vi "U2044XA Measure RF Power.vi"(4 "Route Names":string[](array[string]), 6 "Pwr Mtr Cal":bool=TRUE, 8 "error in":errorcluster, 10 "Input parameters":T1={"Channel (1)"=1, "Avg Count"=4, "Correction Frequency"=50000000.0, "Delay(ms)"=10000, "Reset Device"=FALSE, "ID Query"=FALSE, "Resource Name"="USB0::0x2A8D::0x1E01::MY58390008::INSTR", "Ref Level (dB)"=20.0} {"Ref Level (dB)" format="%^.2e"; "Correction Frequency" format="%.2p"}, 11 "VISA session":refnum<visa-resource-name>="PM2") -> (0 "error out":errorcluster, 2 "dBm":dbl format="%.5f", 3 "dup VISA session":refnum<visa-resource-name>)   [LabVIEW 2015]
doc: "This VI runs one sensor measurement.\n- Open session to sensor specified by Resource Name\n- Sets correct frequency\n- Initialize acqusistion, wait specified time for measurement and reads it."
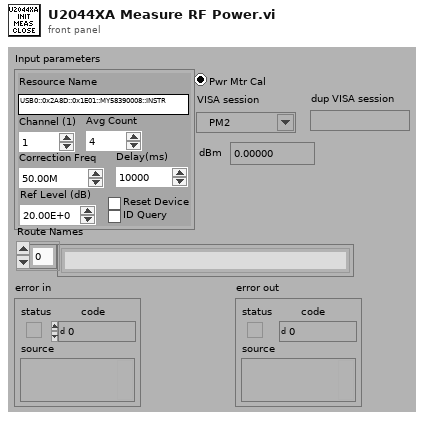
[diagram p1: front panel]
types:
  T1 = cluster{"Channel (1)":i32, "Avg Count":i32, "Correction Frequency":dbl, "Delay(ms)":u32, "Reset Device":bool, "ID Query":bool, "Resource Name":string, "Ref Level (dB)":dbl}
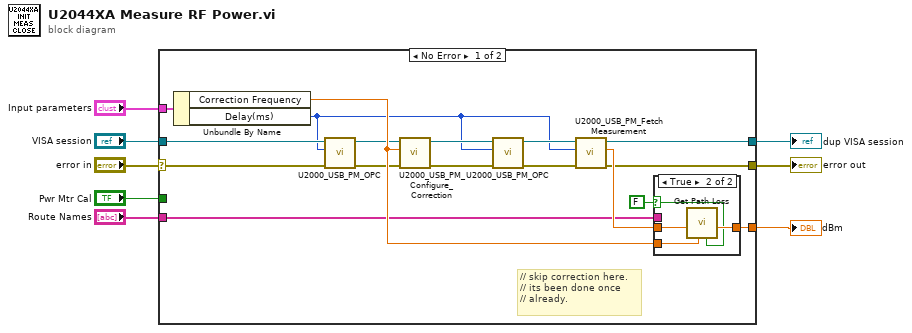
[diagram p0: block diagram]
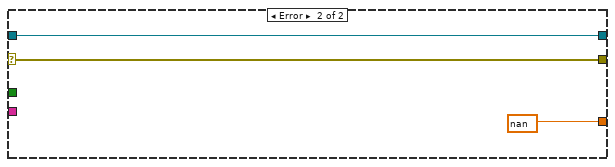
[diagram p3: hidden frame]
diagram:
  n1 = case shown="No Error" "error in" {
    selector: "error in" -> [w16 w33]
    tunnel: [w23 w33] -> w7
    tunnel: "Input parameters" -> [w22 _]
    tunnel: "VISA session" -> [w17 w32]
    tunnel: [w21 w32] -> w4
    tunnel: "Route Names" -> [w20 _]
    tunnel: "Pwr Mtr Cal" -> [_ _]
    tunnel: [w19 nan ("Adjusted Power Level")] -> w1
    frame No Error {
      # "// skip correction here.\n// its been done once\n// already."
      n2 = Unbundle By Name(w22) -> ("Correction Frequency"=w25:dbl, "Delay(ms)"=w9:u32)
      n3 = call "U2000_USB_PM_OPC.vi"("error in (no error)"=w16, "Wait (100ms)"=w9, "VISA resource name"=w17) -> ("error out"=w15:errorcluster, "VISA resource name out"=w14:refnum<visa-resource-name>)  [unwired: 7 in]
      n4 = call "U2000_USB_PM_Configure_Correction.vi"("error in (no error)"=w15, "Frequency (5E+7 Hz)"=w25, "VISA resource name"=w14) -> ("error out"=w13:errorcluster, "VISA resource name out"=w11:refnum<visa-resource-name>)  [unwired: 7 in]
      n5 = call "U2000_USB_PM_OPC.vi"("error in (no error)"=w13, "Wait (100ms)"=w9, "VISA resource name"=w11) -> ("error out"=w12:errorcluster, "VISA resource name out"=w10:refnum<visa-resource-name>)  [unwired: 7 in]
      n6 = call "U2000_USB_PM_Fetch Measurement.vi"("error in (no error)"=w12, "Timeout (10000 ms)"=w9, "VISA resource name"=w10) -> ("error out"=w23:errorcluster, "Measurement"=w24:dbl, "VISA resource name out"=w21:refnum<visa-resource-name>)  [unwired: 6 in]
      n7 = case shown="True" FALSE {
        selector: FALSE -> [_ w27]
        tunnel: w25 -> [_ w28]
        tunnel: w24 -> [w26 w29]
        tunnel: [w26 w30] -> w19
        tunnel: w20 -> [_ _]
        frame False {
        }
        frame True {
          n8 = call "Get Path Loss.vi"("Calibration Enabled"=w27, "Frequency"=w28, "Power Level"=w29) -> ("Adjusted Power Level"=w30:dbl)  [unwired: 4 in, 4 out]
        }
      }
    }
    frame Error {
    }
  }
  "error out" <- w7
  "dup VISA session" <- w4
  "dBm" <- w1
